vi "Confronto_Soglie.vi"(1 "max":dbl, 2 "min":dbl, 3 "distanza":dbl) -> (0 "Comando":i32)   [LabVIEW 2018]
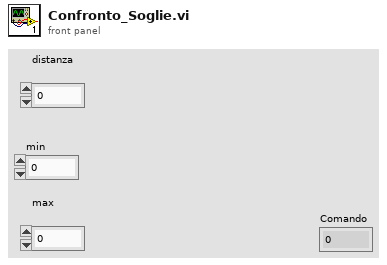
[diagram p1: front panel]
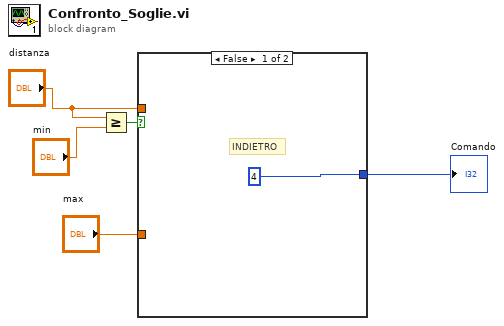
[diagram p0: block diagram]
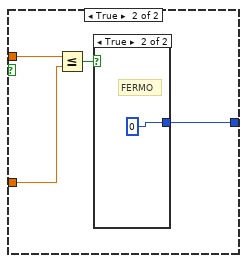
[diagram p2: hidden frame]
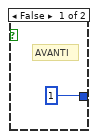
[diagram p3: hidden frame]
diagram:
  n1 = Greater Or Equal?(x="distanza", y="min") -> (x >= y?=w5:bool)
  n2 = case shown="False" w5 {
    tunnel: "distanza" -> [_ w10]
    tunnel: "max" -> [_ w8]
    tunnel: [4 w7] -> w1
    frame False {
      # "INDIETRO"
    }
    frame True {
      n3 = Less Or Equal?(x=w10, y=w8) -> (x <= y?=w9:bool)
      n4 = case shown="True" w9 {
        tunnel: [1 0] -> w7
        frame False {
          # "AVANTI"
        }
        frame True {
          # "FERMO"
        }
      }
    }
  }
  "Comando" <- w1
